vi "Hab Lifter Maintain Position.vi"(7 "Description":string, 8 "Command Info In":T1, 11 "Both?":bool) -> (0 "Command Info Out":T1)   [LabVIEW 2018]
doc: "This template includes code for deadband comparision to avoid excessive command scheduling. It is particularly useful for joystick-driven commands.\n\nBe sure to right-click and select New from Template and save with a new command name."
uses:
  <vilib>/Rock Robotics/WPI/Framework/Command Status Info.ctl
  <vilib>/Rock Robotics/WPI/Framework/Completion Status.ctl
  <vilib>/Rock Robotics/WPI/Framework/Completion Notifier.ctl
  Implementation/Hab Lifter Setpoints.ctl
  Implementation/Hab Lifter Operations.ctl
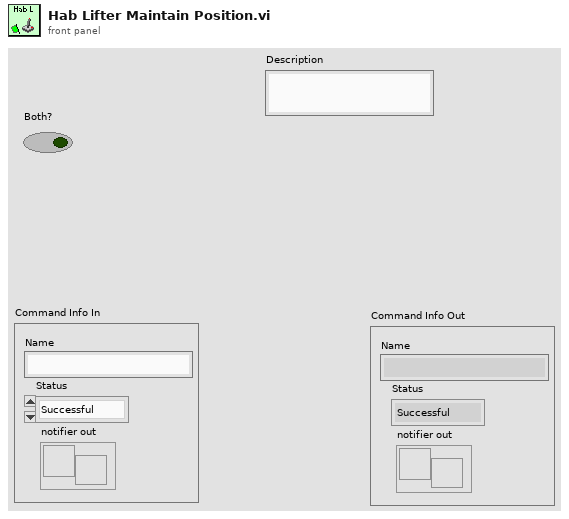
[diagram p1: front panel]
types:
  T1 = typedef "Command Status Info.ctl" = cluster{"Name":string, "Status":T2, "notifier out":T3}
  T2 = typedef "Completion Status.ctl" = enum16{"Successful", "Aborted", "Incomplete"}
  T3 = typedef "Completion Notifier.ctl" = refnum<notifier>
  T4 = typedef "Hab Lifter Setpoints.ctl" = cluster{"Operation":T5, "Left Setpoint":dbl, "Right Setpoint":dbl, "PID Position":i16}
  T5 = typedef "Hab Lifter Operations.ctl" = enum16{"Reserve", "Read Current", "Immediate", "Immediate Simultaneous", "Yeah It's PID", "Maintain Both", "Maintain Back"}
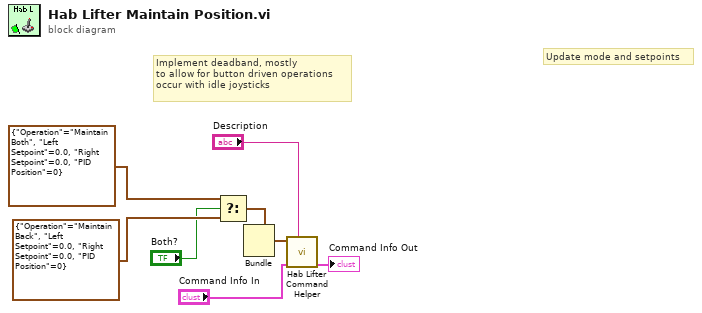
[diagram p0: block diagram]
diagram:
  # "Implement deadband, mostly\nto allow for button driven operations\noccur with idle joysticks"
  # "Update mode and setpoints"
  n1 = Select(t=T4 {"Operation"=enum."Maintain Both", "Left Setpoint"=0.0, "Right Setpoint"=0.0, "PID Position"=0} ("SubSystem Data"), s="Both?", f=T4 {"Operation"=enum."Maintain Back", "Left Setpoint"=0.0, "Right Setpoint"=0.0, "PID Position"=0} ("SubSystem Data")) -> (s? t:f=w4:T4)
  n2 = Bundle(cluster=w4) -> (w5:T4)  [unwired: 4 in]
  n3 = call "Hab Lifter Command Helper.vi"("Description"="Description", "Command Info In"="Command Info In", "SubSystem Data"=w5) -> ("Command Info Out"=→"Command Info Out":T1)  [unwired: 6 in, 2 out]
